vi "Integer Check Array.vi"(11 "Array":u8[](array[numeric])) -> (3 "Error":bool)   [LabVIEW 2015, in "Sudoku Library.lvlib"]
doc: "Created IvanLis by LabVIEW Portal\nProfile: http://labviewportal.org/memberlist.php?mode=viewprofile&u=987\neMail: IvanLisanov@gMail.com\nTelegram: https://t.me/IvanLis"
uses:
  Sudoku Library.lvlib
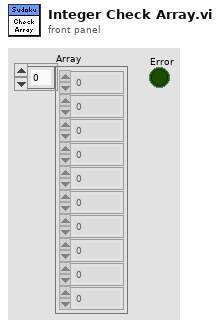
[diagram p1: front panel]
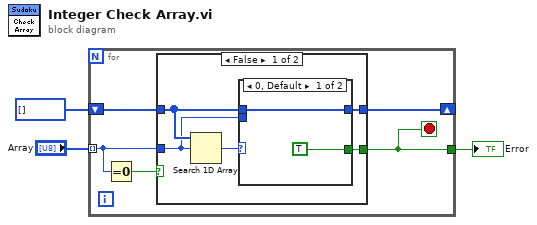
[diagram p0: block diagram]
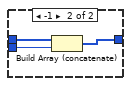
[diagram p2: hidden frame]
diagram:
  n1 = for {
    shift-right: [w6] -> _
    shift-left: u8[] [] -> [w7]
    tunnel: "Array" -> [w5] mode=indexing
    tunnel: [w4] -> w2
    stop <- w4 stop-if-true
    n2 = Equal To 0?(x=w5) -> (x = 0?=w8:bool)
    n3 = case shown="False" w8 {
      tunnel: w7 -> [w11 w19]
      tunnel: [w10 w19] -> w6
      tunnel: w5 -> [w9 _]
      tunnel: [w12 _] -> w4
      frame False {
        n4 = Search 1D Array(1D array=w11, element=w9) -> (index of element=w13:i32)  [unwired: 1 in]
        n5 = case shown="0, Default" w13 {
          tunnel: [TRUE _] -> w12
          tunnel: w11 -> [w14 w18]
          tunnel: [w14 w17] -> w10
          tunnel: w9 -> [_ w16]
          frame 0, Default {
          }
          frame -1 {
            n6 = Build Array (concatenate)(w18, w16) -> (w17:u8[])
          }
        }
      }
      frame True {
      }
    }
  }
  "Error" <- w2
